vi "Test.vi"() -> ()   [LabVIEW 2019]
uses:
  Queued Listbox.xctl
panel:
  out "Queued Listbox ref":refnum<vi>
  out "Button press item":string
  in  "Stop Button":bool
  in  "Selections":string[](array[string])=["Two", "3"]
  out "Selections out":string[](array[string])=["asd", "ads"]
  out "error out":errorcluster
  in  "Items":string[](array[string])=["Uno", "Two", "3"]
  in  "Queued Listbox":string[](xcontrol)=["asd", "ads"]
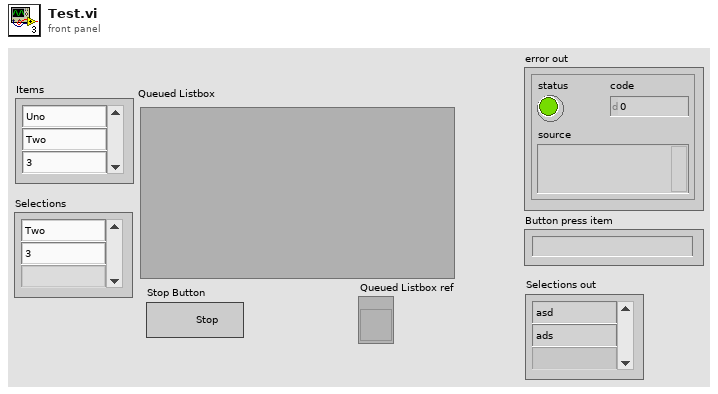
[diagram p1: front panel]
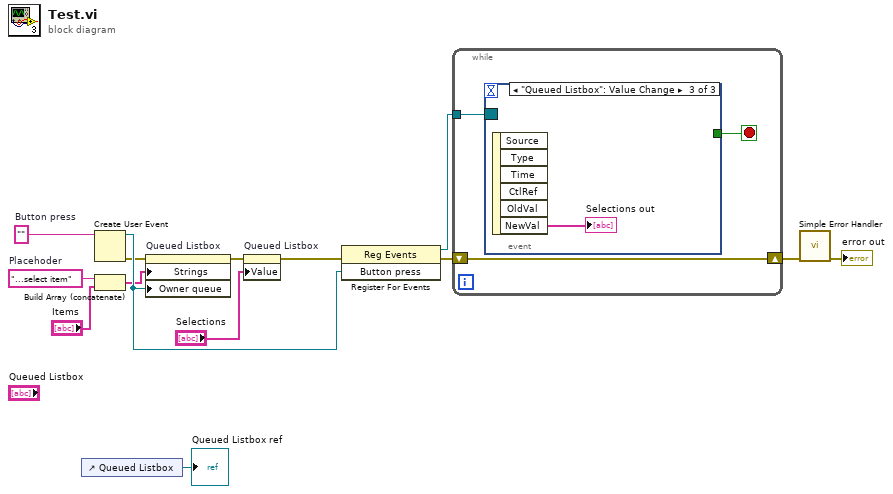
[diagram p0: block diagram]
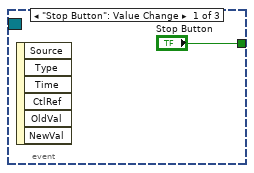
[diagram p2: hidden frame]
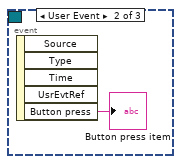
[diagram p3: hidden frame]
diagram:
  w3 = "...select item"  # Placehoder
  w11 = ""  # Button press
  n1 = control-ref of="Queued Listbox"() -> (→"Queued Listbox ref":refnum<vi>)
  n2 = Create User Event(user event datatype=w11) -> (user event=w10:refnum<user-event>, error out=w9:errorcluster)  [unwired: 1 in]
  n3 = Build Array (concatenate)(w3, "Items") -> (w4:string[])
  n4 = property on="Queued Listbox" class="Queued Listbox (strict)"(error in=w9, "Strings"=w4, "Owner queue"=w10) -> (error out=w14:errorcluster)  [unwired: 1 in, 1 out]
  n5 = property on="Queued Listbox" class="Queued Listbox (strict)"(error in=w14, "Value"="Selections") -> (error out=w8:errorcluster)  [unwired: 1 in, 1 out]
  n6 = register-events(error in=w8, w10) -> (reference out=w7:refnum<event-registration>, error out=w6:errorcluster)  [unwired: 1 in]
  n7 = while {
    tunnel: w7 -> [w16]
    shift-right: [w15] -> w2
    shift-left: w6 -> [w15]
    stop <- w17 stop-if-true
    n8 = event shown="[2] \"Queued Listbox\": Value Change" {
      selector: w16 -> [_ _ _]
      dyn-events: _ -> [_ _ _]
      timeout: _ -> [_ _ _]
      tunnel: ["Stop Button" _ _] -> w17
      event "Stop Button": Value Change {
        n9 = event-data() -> ()  [unwired: 1 in, 6 out]
      }
      event User Event {
        n10 = event-data() -> ("Button press"=→"Button press item":string)  [unwired: 1 in, 4 out]
      }
      event "Queued Listbox": Value Change {
        n11 = event-data() -> ("NewVal"=→"Selections out":string[])  [unwired: 1 in, 5 out]
      }
    }
  }
  n12 = call <vilib>:"Simple Error Handler.vi"("error in (no error)"=w2) -> ("error out"=→"error out":errorcluster)  [unwired: 4 in, 4 out]
